vi "Ring Buffer CH1 short rev2.vi"(9 "Index":i32=188, 10 "Profiles to Average":i32=30, 11 "Input Array":dbl[](array[numeric])) -> (1 "AvgArray":dbl[](array[numeric]), 3 "RingBufferOut":dbl[][](array[numeric]))   [LabVIEW 2012]
panel:
  out "RingArraySize":dbl[](array[numeric])=[30.0, 559.0]
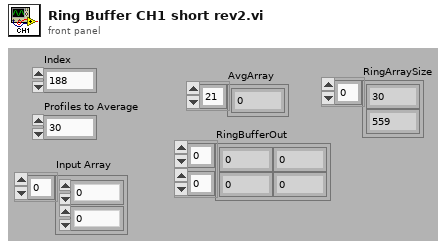
[diagram p1: front panel]
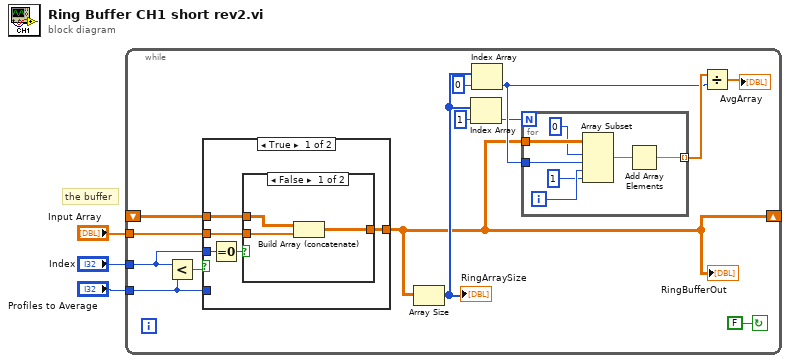
[diagram p0: block diagram]
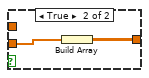
[diagram p2: hidden frame]
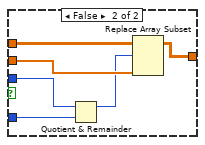
[diagram p3: hidden frame]
diagram:
  # "the buffer"
  n1 = while {
    shift-right: [w4] -> _
    shift-left: _ -> [w13]
    tunnel: "Profiles to Average" -> [w9]
    tunnel: "Index" -> [w15]
    tunnel: "Input Array" -> [w14]
    stop <- FALSE ("stop") continue-if-true
    n2 = Less?(x=w15, y=w9) -> (x < y?=w16:bool)
    n3 = case shown="True" w16 {
      tunnel: w15 -> [w25 w40]
      tunnel: [w26 w36] -> w4
      tunnel: w9 -> [_ w39]
      tunnel: w14 -> [w27 w37]
      tunnel: w13 -> [w28 w38]
      frame True {
        n4 = Equal To 0?(x=w25) -> (x = 0?=w29:bool)
        n5 = case shown="False" w29 {
          tunnel: [w30 w34] -> w26
          tunnel: w28 -> [w32 _]
          tunnel: w27 -> [w31 w33]
          frame False {
            n6 = Build Array (concatenate)(w32, w31) -> (w30:dbl[][])
          }
          frame True {
            n7 = Build Array(w33) -> (w34:dbl[][])
          }
        }
      }
      frame False {
        n8 = Quotient & Remainder(x=w40, y=w39) -> (x-y*floor(x/y)=w35:i32)  [unwired: 1 out]
        n9 = Replace Array Subset(array=w38, new element=w37, index (row)=w35) -> (w36:dbl[][])  [unwired: 1 in]
      }
    }
    "RingBufferOut" <- w4
    n10 = Array Size(array=w4) -> (size(s)=w8:i32[])
    "RingArraySize" <- w8
    n11 = Index Array(array=w8, index=1) -> (element=w5:i32)
    n12 = Index Array(array=w8, index=0) -> (element=w6:i32)
    n13 = for {
      N: w5 -> [_]
      tunnel: [w19] -> w10 mode=indexing
      tunnel: w6 -> [w24]
      tunnel: w4 -> [w23]
      i -> [w21]
      n14 = Array Subset(array=w23, index (row)=0, length (row)=w24, index (col)=w21, length (col)=1 ("length")) -> (w22:dbl[][])
      n15 = Add Array Elements(numeric array=w22) -> (sum=w19:dbl)
    }
    n16 = Divide(x=w10, y=w6) -> (x/y=→"AvgArray":dbl[])
  }
